vi "Validation.vi"(10 "Array":refnum<vi>[](array[refnum]), 11 "Array 2":refnum<vi>[](array[refnum])) -> (3 "empty?":bool)   [LabVIEW 2013]
uses:
  <userlib>/_OpenG.lib/array/array.llb/Filter 1D Array (String)__ogtk.vi
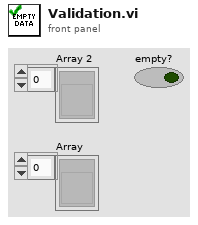
[diagram p1: front panel]
types:
  T1 = typedef "ComboBox.ctl" = string
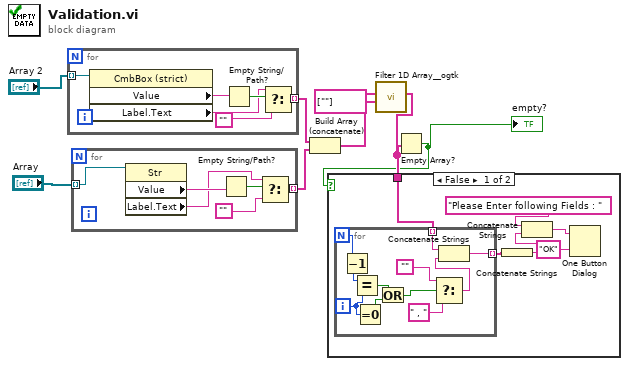
[diagram p0: block diagram]
diagram:
  n1 = for {
    tunnel: "Array 2" -> [w14] mode=indexing
    tunnel: [w10] -> w4 mode=indexing
    n2 = property class="CmbBox (strict)"(reference=w14) -> ("Value"=w13:T1, "Label.Text"=w11:string)  [unwired: 1 in, 2 out]
    n3 = Empty String/Path?(string/path=w13) -> (empty?=w12:bool)
    n4 = Select(t=w11, s=w12, f="") -> (s? t:f=w10:string)
  }
  n5 = for {
    tunnel: "Array" -> [w20] mode=indexing
    tunnel: [w16] -> w3 mode=indexing
    n6 = property class="Str"(reference=w20) -> ("Value"=w18:string, "Label.Text"=w17:string)  [unwired: 1 in, 2 out]
    n7 = Empty String/Path?(string/path=w18) -> (empty?=w19:bool)
    n8 = Select(t=w17, s=w19, f="") -> (s? t:f=w16:string)
  }
  n9 = Build Array (concatenate)(w4, w3) -> (w6:string[])
  n10 = call-poly <userlib>:"Filter 1D Array__ogtk.vi"("items to filter"=string[] [""], "array"=w6) -> ("filtered array"=w8:string[])  [unwired: 4 in, 1 out]
  n11 = Empty Array?(array=w8) -> (empty?=w5:bool)
  "empty?" <- w5
  n12 = case shown="False" w5 {
    tunnel: w8 -> [w21 _]
    frame False {
      n13 = for {
        N -> [w32]
        tunnel: w21 -> [w37] mode=indexing
        tunnel: [w36] -> w23 mode=indexing
        i -> [w31]
        n14 = Decrement(x=w32) -> (x-1=w30:i32)
        n15 = Equal?(x=w30, y=w31) -> (x = y?=w29:bool)
        n16 = Equal To 0?(x=w31) -> (x = 0?=w28:bool)
        n17 = Or(x=w29, y=w28) -> (x .or. y?=w27:bool)
        n18 = Select(t="", s=w27, f=" , ") -> (s? t:f=w33:string)
        n19 = Concatenate Strings(w37, w33) -> (w36:string)
      }
      n20 = Concatenate Strings(w23) -> (w22:string)
      n21 = Concatenate Strings("Please Enter following Fields : ", w22) -> (w24:string)
      n22 = One Button Dialog(message=w24, button name ("OK")="OK") -> ()  [unwired: 1 out]
    }
    frame True {
    }
  }
